vi "Get.vi"(8 "error in (no error)":errorcluster, 9 "Name":string, 11 "LV Argument Parser in":refnum<class "LV Argument Parser.lvclass">) -> (0 "error out":errorcluster, 1 "element":variant, 2 "key not found?":bool, 3 "LV Argument Parser out":refnum<class "LV Argument Parser.lvclass">)   [LabVIEW 2023, in "LV ArgParse.lvlib" / "LV Argument Parser.lvclass"]
uses:
  LV Argument Parser.lvclass
  LV Argument Parser.lvclass/LV Argument Parser.ctl
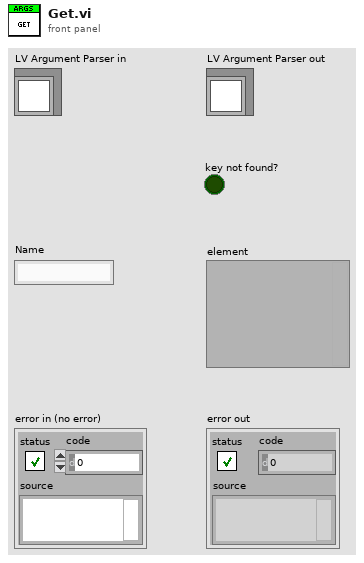
[diagram p1: front panel]
types:
  T1 = typedef "LV ArgParse.lvlib/LV Argument Parser.lvclass/Argument Definition.ctl" = cluster{"Name":string, "short (positional)":string, "long (positional)":string, "action":enum16{"store", "store-const", "store-false", "store-true", "append", "append-const", "count", "help", "version"}, "choices":string[], "const":string, "default":string, "dest (=name)":string, "help":string, "Number":i32, "Required":bool, "Type":enum16{"String", "Int", "Uint", "Float", "Bool", "Date", "Path"}}
  T2 = enum16{"store", "store-const", "store-false", "store-true", "append", "append-const", "count", "help", "version"}
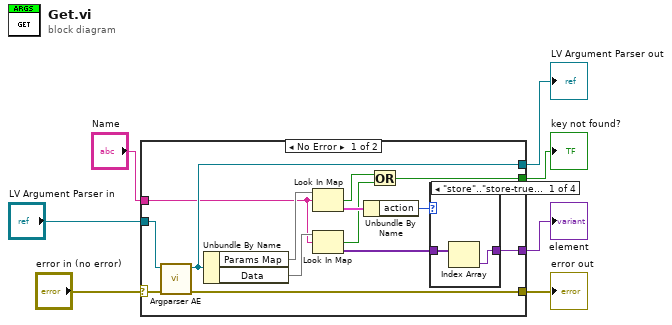
[diagram p0: block diagram]
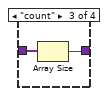
[diagram p3: hidden frame]
diagram:
  n1 = case shown="No Error" "error in (no error)" {
    selector: "error in (no error)" -> [w21 w28]
    tunnel: [w20 w28] -> w6
    tunnel: [w18 w27] -> w4
    tunnel: "LV Argument Parser in" -> [w19 w27]
    tunnel: "Name" -> [w15 _]
    tunnel: [w11 _] -> w2
    tunnel: [w9 _] -> w1
    frame No Error {
      n2 = call "Argparser AE.vi"("error in (no error)"=w21, "LV Argument Parser in"=w19) -> ("error out"=w20:errorcluster, "LV Argument Parser out"=w18:refnum<class "LV Argument Parser.lvclass">)  [unwired: 8 in]
      n3 = Unbundle By Name(w18) -> ("Params Map"=w16:map{string, T1}, "Data"=w17:map{string, variant[]})
      n4 = Look In Map(map=w16, key=w15) -> (key not found?=w8:bool, value=w14:T1)  [unwired: 1 in]
      n5 = Look In Map(map=w17, key=w15) -> (key not found?=w10:bool, value=w12:variant[])  [unwired: 1 in]
      n6 = Unbundle By Name(w14) -> ("action"=w13:T2)
      n7 = Or(x=w8, y=w10) -> (x .or. y?=w9:bool)
      n8 = case shown="\"store\"..\"store-true\"" w13 {
        tunnel: w12 -> [w23 w24 w26 _]
        tunnel: [w22 w24 w25 _] -> w11
        frame "store".."store-true" {
          n9 = Index Array(array=w23) -> (element=w22:variant)  [unwired: 1 in]
        }
        frame "append", "append-const" {
        }
        frame "count" {
          n10 = Array Size(array=w26) -> (size(s)=w25:i32)
        }
        frame Default {
        }
      }
    }
    frame Error {
    }
  }
  "error out" <- w6
  "LV Argument Parser out" <- w4
  "element" <- w2
  "key not found?" <- w1
